vi "TreeNode Update Segment.vi"(0 "TreeNode DVR in":refnum<data-value>, 1 "Start":refnum<data-value>, 2 "End":refnum<data-value>, 3 "Dimension":refnum<data-value>, 5 "error in (no error)":errorcluster) -> (14 "TreeNode DVR out":refnum<data-value>, 19 "error out":errorcluster)   [LabVIEW 2015, in "MDSplus.lvlib"]
uses:
  <userlib>/MDSplus/Library/MDSplus.lvlib
  <userlib>/MDSplus/Classes/Data_Class/TreeNode_Class/TreeNode.lvclass
  <userlib>/MDSplus/Classes/Data_Class/Data.lvclass
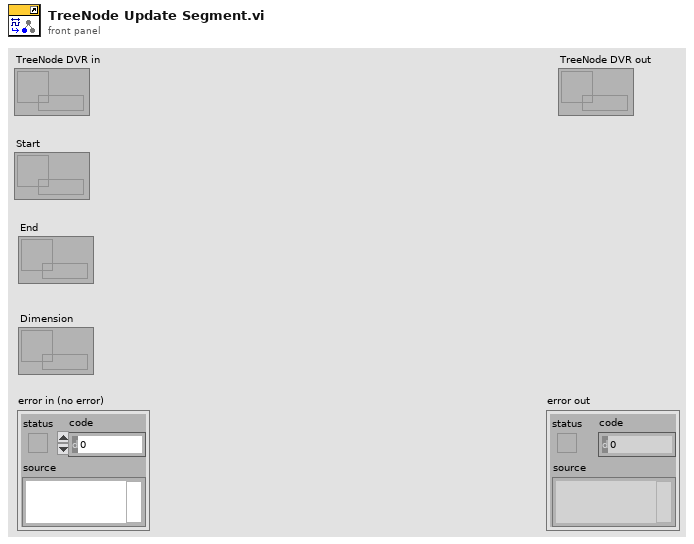
[diagram p1: front panel]
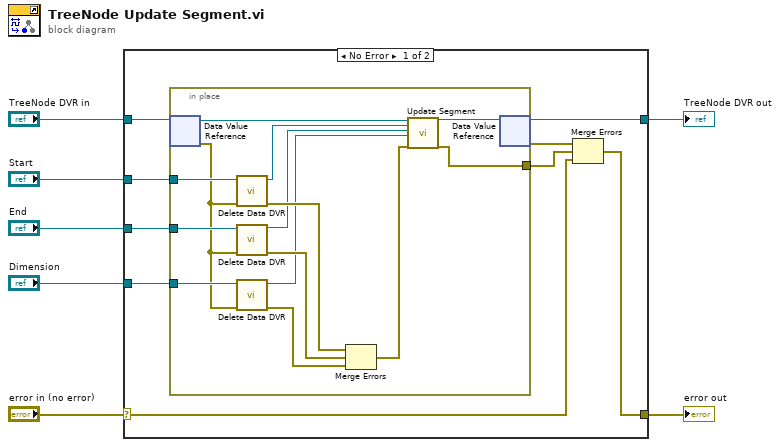
[diagram p0: block diagram]
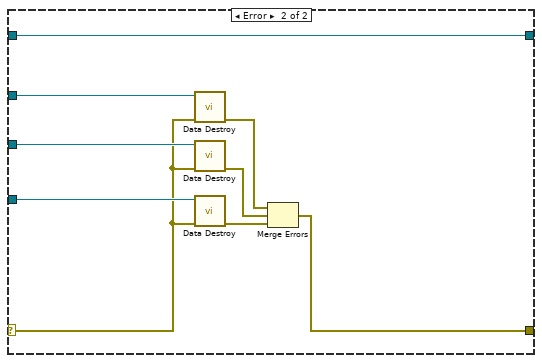
[diagram p2: hidden frame]
diagram:
  n1 = case shown="No Error" "error in (no error)" {
    selector: "error in (no error)" -> [w11 w32]
    tunnel: [w10 w33] -> w7
    tunnel: [w9 w31] -> w5
    tunnel: "Start" -> [w16 w39]
    tunnel: "End" -> [w15 w38]
    tunnel: "Dimension" -> [w14 w37]
    tunnel: "TreeNode DVR in" -> [w13 w31]
    frame No Error {
      n2 = in-place {
        in-place-border: w16 -> [w30]
        in-place-border: w15 -> [w29]
        in-place-border: w14 -> [w28]
        in-place-border: [w20] -> w8
        n3 = in-place-dvr #1(w13) -> (w23:refnum<class "TreeNode.lvclass">, w24:errorcluster)
        n4 = call <userlib>:"Delete Data DVR.vi"("error in (no error)"=w24, "Data DVR in"=w30) -> ("error out"=w25:errorcluster, "Data out"=w19:refnum<class "Data.lvclass">)  [unwired: 8 in]
        n5 = call <userlib>:"Delete Data DVR.vi"("error in (no error)"=w24, "Data DVR in"=w29) -> ("error out"=w26:errorcluster, "Data out"=w18:refnum<class "Data.lvclass">)  [unwired: 8 in]
        n6 = call <userlib>:"Delete Data DVR.vi"("error in (no error)"=w24, "Data DVR in"=w28) -> ("error out"=w27:errorcluster, "Data out"=w17:refnum<class "Data.lvclass">)  [unwired: 8 in]
        n7 = Merge Errors(w25, w26, w27) -> (w21:errorcluster)
        n8 = call <userlib>:"Update Segment.vi"("TreeNode in"=w23, "Start"=w19, "End"=w18, "Dimension"=w17, "error in (no error)"=w21) -> ("TreeNode out"=w22:refnum<class "TreeNode.lvclass">, "error out"=w20:errorcluster)  [unwired: 13 in]
        n9 = in-place-dvr #1(w22) -> (w9:refnum<data-value>, w12:errorcluster)
      }
      n10 = Merge Errors(w12, w8, w11) -> (w10:errorcluster)
    }
    frame Error {
      n11 = call <userlib>:"Data Destroy.vi"("error in (no error)"=w32, "Data DVR in"=w39) -> ("error out"=w36:errorcluster)  [unwired: 9 in]
      n12 = call <userlib>:"Data Destroy.vi"("error in (no error)"=w32, "Data DVR in"=w38) -> ("error out"=w35:errorcluster)  [unwired: 9 in]
      n13 = call <userlib>:"Data Destroy.vi"("error in (no error)"=w32, "Data DVR in"=w37) -> ("error out"=w34:errorcluster)  [unwired: 9 in]
      n14 = Merge Errors(w36, w35, w34) -> (w33:errorcluster)
    }
  }
  "error out" <- w7
  "TreeNode DVR out" <- w5
